vi "Create Instance Impl.vi"(8 "error in (no error)":errorcluster, 10 "Fluidics Configuration":T1={"Serial Port"="COM3", "Device Type"=enum."Disabled"}, 11 "Simulated Autosampler in":refnum<class "Simulated Autosampler.lvclass">) -> (0 "error out":errorcluster, 3 "Simulated Autosampler out":refnum<class "Simulated Autosampler.lvclass">)   [LabVIEW 2023, in "Simulated Autosampler.lvlib" / "Simulated Autosampler.lvclass"]
uses:
  Simulated Autosampler.lvclass
  Resources/Type Defs/Autosampler Configuration.ctl
  Autosampler/Autosampler Status.ctl
  Autosampler/Autosampler State.ctl
  Simulated Autosampler.lvclass/Simulated Autosampler.ctl
  Autosampler/Autosampler.lvlib
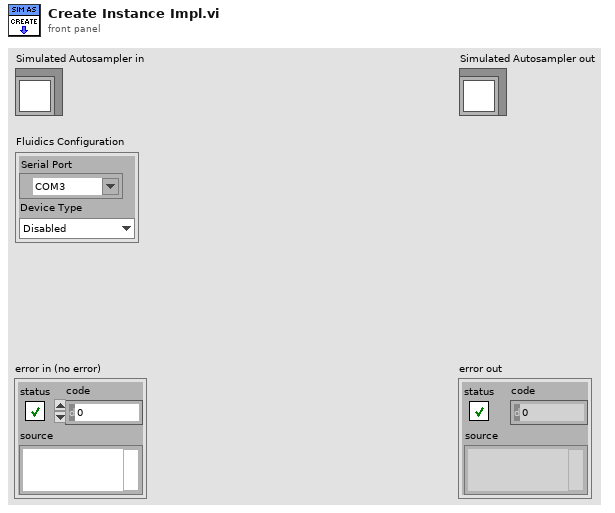
[diagram p1: front panel]
types:
  T1 = typedef "Autosampler Configuration.ctl" = cluster{"Serial Port":refnum<visa-resource-name>, "Device Type":enum16{"Disabled", "Simulate", "Alltesta"}}
  T2 = typedef "Autosampler.lvlib/Autosampler Status.ctl" = cluster{"State":T3, "Valve Position":u16, "Well index":u16, "Fill Volume":u16, "Needle Position":enum16{"Home", "Well", "Wash Port"}}
  T3 = typedef "Autosampler.lvlib/Autosampler State.ctl" = enum16{"Ready", "Injection", "Washing", "Shaking", "Getting Ready", "Error"}
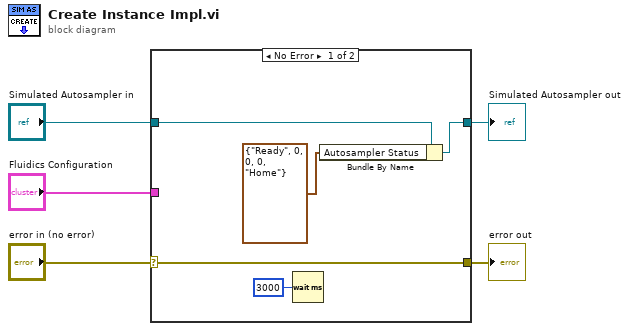
[diagram p0: block diagram]
diagram:
  n1 = case shown="No Error" "error in (no error)" {
    selector: "error in (no error)" -> [w10 w11]
    tunnel: [w10 w11] -> w4
    tunnel: "Simulated Autosampler in" -> [w9 w12]
    tunnel: [w8 w12] -> w2
    tunnel: "Fluidics Configuration" -> [_ _]
    frame No Error {
      n2 = Wait (ms)(milliseconds to wait=u32 3000) -> ()  [unwired: 1 out]
      n3 = Bundle By Name(cluster=w9, "Autosampler Status"=T2 {"State"=enum."Ready", "Valve Position"=0, "Well index"=0, "Fill Volume"=0, "Needle Position"=enum."Home"}) -> (w8:refnum<class "Simulated Autosampler.lvclass">)
    }
    frame Error {
    }
  }
  "error out" <- w4
  "Simulated Autosampler out" <- w2
